vi "Save-to-hp_state.vi"(8 "hp_state_in (u64)":u64[](array[numeric]) format="%.0x", 9 "hp_state_in in":u8[](array[numeric]) format="%.0x", 10 "j":u64, 11 "New-Val":u64[](array[numeric]) format="%.0x") -> (2 "hp_state_out (u64)":u64[](array[numeric]) format="%.0x", 3 "hp_state_in out":u8[](array[numeric]) format="%.0x")   [LabVIEW 2017]
panel:
  out "j/8":u64
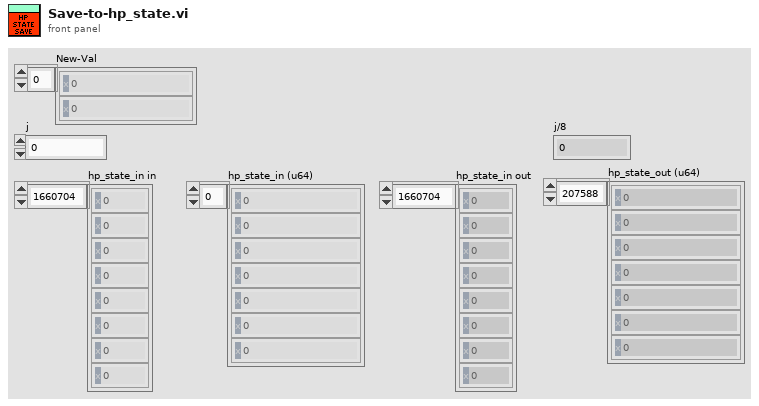
[diagram p1: front panel]
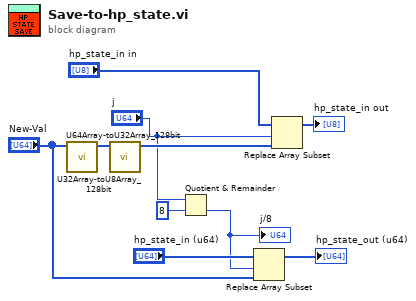
[diagram p0: block diagram]
diagram:
  n1 = call "U64Array-toU32Array_128bit.vi"("2 x U64"="New-Val") -> ("4 x U32"=w9:u32[])  [unwired: 10 in]
  n2 = call "U32Array-toU8Array_128bit.vi"("4 x U32"=w9) -> ("16 x U8"=w10:u8[])  [unwired: 10 in]
  n3 = Quotient & Remainder(x="j", y=u64 8) -> (floor(x/y)=w3:u64)  [unwired: 1 out]
  "j/8" <- w3
  n4 = Replace Array Subset(array="hp_state_in (u64)", new element="New-Val", index=w3) -> (→"hp_state_out (u64)":u64[])
  n5 = Replace Array Subset(array="hp_state_in in", new element=w10, index="j") -> (→"hp_state_in out":u8[])
